vi "[[Boolean]] to [[1,NaN]] (SGL).vi"(1 "Valid?":bool[][](array[boolean])) -> (2 "# Valid":i32, 4 "1 or NaN Array":sgl[][](array[numeric]))   [LabVIEW 2021, in "Arrays.lvlib"]
uses:
  Arrays.lvlib
  Utilities/Utilities.lvlib
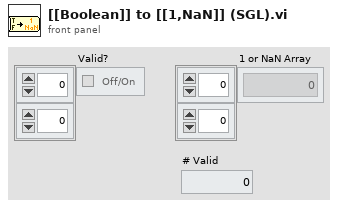
[diagram p1: front panel]
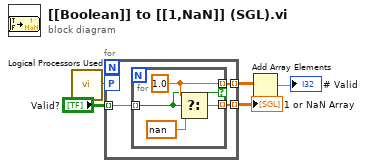
[diagram p0: block diagram]
diagram:
  n1 = call "Logical Processors Used.vi"() -> ("# Logical Processor Used"=w1:i32)  [unwired: 6 in]
  n2 = for {
    tunnel: "Valid?" -> [w8] mode=indexing
    workers-P: w1 -> [_]
    tunnel: [w7] -> w4 mode=indexing
    tunnel: [w6] -> w3 mode=indexing
    n3 = for {
      tunnel: w8 -> [w9] mode=indexing
      tunnel: [w12] -> w7 mode=indexing
      tunnel: [w10] -> w6 mode=indexing if=w9
      w10 = sgl 1.0 ("t")
      n4 = Select(t=w10, s=w9, f=sgl nan) -> (s? t:f=w12:sgl)
    }
  }
  "1 or NaN Array" <- w4
  n5 = Add Array Elements(numeric array=w3) -> (sum=→"# Valid":sgl)
